vi "Set Front Panel Properties.vi"(3 "Water Flow Graph Refnum":refnum<vi>, 5 "Wash Op Refnum":refnum<vi>, 7 "Car Slider Refnum":refnum<vi>, 8 "error in (no error)":errorcluster, 9 "Control":T1(ring), 10 "DtCy Slider Refnum":refnum<vi>, 11 "Start Refnum":refnum<vi>) -> (0 "error out":errorcluster)   [LabVIEW 2021]
doc: "This VI sets the front panel properties to the ''enabled'' or ''disabled and grayed out'' state."
uses:
  Controls/Wash Options.ctl
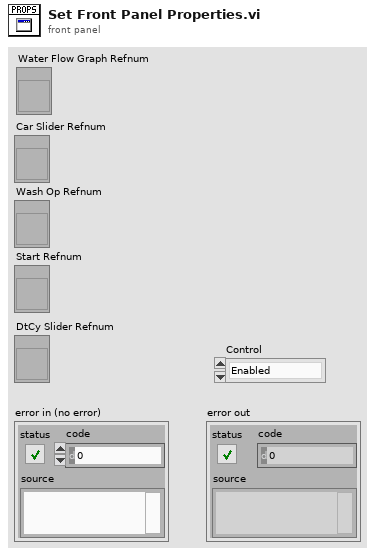
[diagram p1: front panel]
types:
  T1 = enum8{"Enabled", "Disabled", "Disabled and Grayed Out"}
  T2 = enum16{"Always On", "Always Off", "Off While Running"}
  T3 = typedef "Wash Options.ctl" = cluster{"Underbody Wash":bool, "Bug Remover":bool, "Pre-Soak":bool, "High Pressure Wash":bool, "Low Pressure Wax":bool, "Spot Free Rinse":bool, "Tire Shine Foam":bool, "Air Dry":bool}
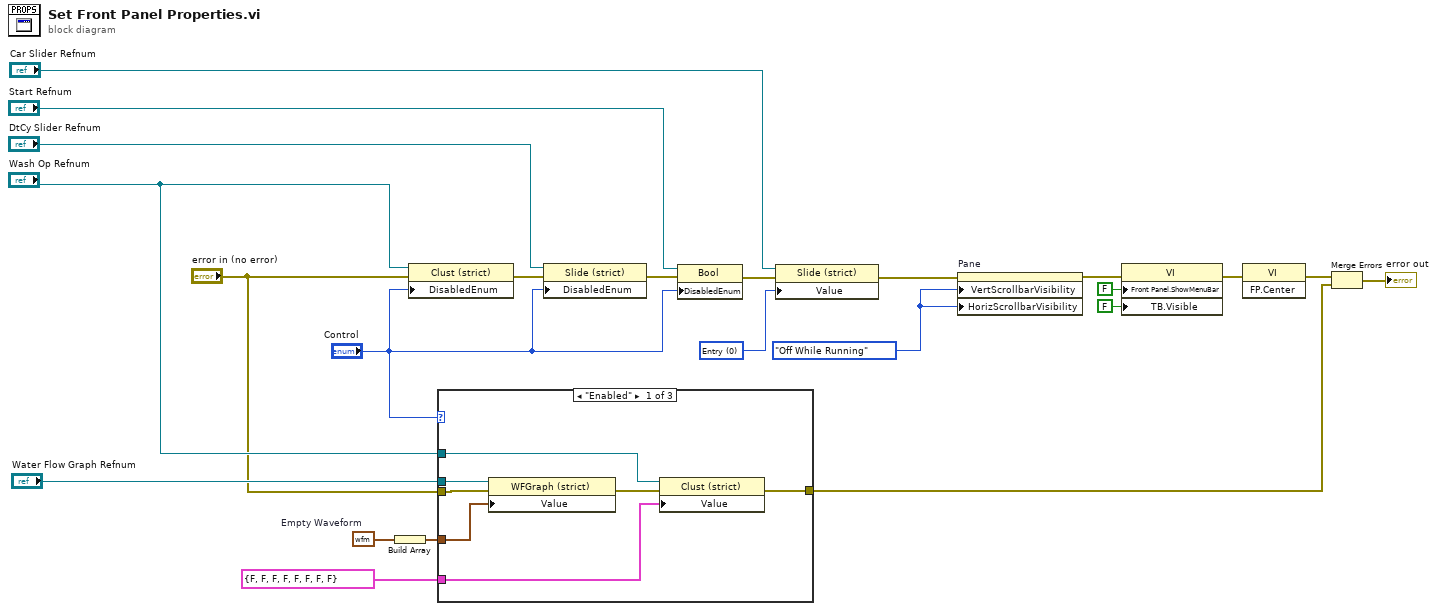
[diagram p0: block diagram]
diagram:
  w12 = T2."Off While Running" ("Vertical Scrollbar Visibility")
  w15 = waveform(dbl) {"t0"=timestamp(0 s since 1904-01-01), "dt"=1.0, "Y"=[]}  # Empty Waveform
  w23 = u8 0 items=["Entry", "Station 1", "Station 2", "Station 3", "Exit"] ("Car Position Slider")
  n1 = Build Array(w15) -> (w16:waveform(dbl)[])
  n2 = property on="Property Node" class="Clust (strict)"(reference="Wash Op Refnum", error in="error in (no error)", "DisabledEnum"="Control") -> (error out=w22:errorcluster)  [unwired: 1 out]
  n3 = case shown="\"Enabled\"" "Control" {
    tunnel: w16 -> [w30 _ _]
    tunnel: "Water Flow Graph Refnum" -> [w29 _ _]
    tunnel: "Wash Op Refnum" -> [w27 _ _]
    tunnel: T3 {"Underbody Wash"=FALSE, "Bug Remover"=FALSE, "Pre-Soak"=FALSE, "High Pressure Wash"=FALSE, "Low Pressure Wax"=FALSE, "Spot Free Rinse"=FALSE, "Tire Shine Foam"=FALSE, "Air Dry"=FALSE} ("Wash Options") -> [w26 _ _]
    tunnel: "error in (no error)" -> [w25 w31 w32]
    tunnel: [w24 w31 w32] -> w2
    frame "Enabled" {
      n4 = property on="Property Node" class="WFGraph (strict)"(reference=w29, error in=w25, "Value"=w30) -> (error out=w28:errorcluster)  [unwired: 1 out]
      n5 = property on="Property Node" class="Clust (strict)"(reference=w27, error in=w28, "Value"=w26) -> (error out=w24:errorcluster)  [unwired: 1 out]
    }
    frame "Disabled" {
    }
    frame "Disabled and Grayed Out" {
    }
  }
  n6 = property on="Property Node" class="Slide (strict)"(reference="DtCy Slider Refnum", error in=w22, "DisabledEnum"="Control") -> (error out=w21:errorcluster)  [unwired: 1 out]
  n7 = property on="Property Node" class="Bool"(reference="Start Refnum", error in=w21, "DisabledEnum"="Control") -> (error out=w17:errorcluster)  [unwired: 1 out]
  n8 = property on="Property Node" class="Slide (strict)"(reference="Car Slider Refnum", error in=w17, "Value"=w23) -> (error out=w7:errorcluster)  [unwired: 1 out]
  n9 = property on="Pane" class="Pane"(error in=w7, "VertScrollbarVisibility"=w12, "HorizScrollbarVisibility"=w12) -> (error out=w9:errorcluster)  [unwired: 1 in, 1 out]
  n10 = property class="VI"(error in=w9, "Front Panel.ShowMenuBar"=FALSE ("Front Panel Window:Show Menu Bar"), "TB.Visible"=FALSE ("Tool Bar:Visible")) -> (error out=w8:errorcluster)  [unwired: 1 in, 1 out]
  n11 = invoke class="VI" method="FP.Center"(error in=w8) -> (error out=w3:errorcluster)  [unwired: 2 in, 2 out]
  n12 = Merge Errors(w3, w2) -> (→"error out":errorcluster)
